vi "SP Sort Limit Points by Frequency.vi"(4 "Points":T1[](array[typedef])) -> (1 "Sorted Points":T1[](array[typedef]))   [LabVIEW 2011]
uses:
  TypeDefs/SP Limit Point.ctl
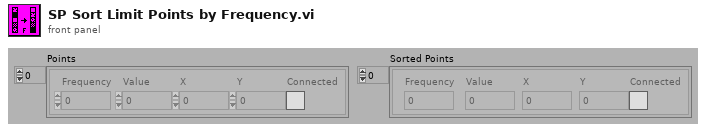
[diagram p1: front panel]
types:
  T1 = typedef "SP Limit Point.ctl" = cluster{"Frequency":dbl, "Value":dbl, "X":dbl, "Y":dbl, "Connected":bool}
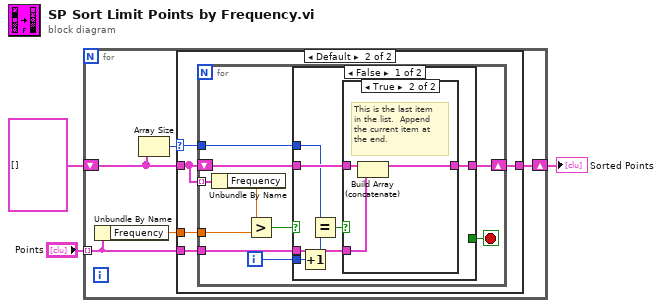
[diagram p0: block diagram]
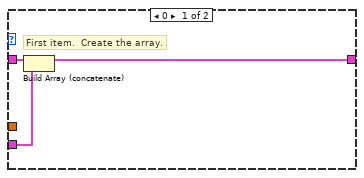
[diagram p2: hidden frame]
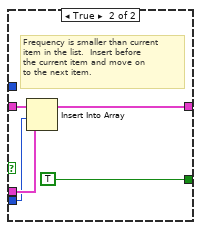
[diagram p4: hidden frame]
diagram:
  n1 = for {
    tunnel: "Points" -> [w6] mode=indexing
    shift-right: [w7] -> w2
    shift-left: T1[] [] ("Points") -> [w8]
    n2 = Unbundle By Name(w6) -> ("Frequency"=w5:dbl)
    n3 = Array Size(array=w8) -> (size(s)=w4:i32)
    n4 = case shown="Default" w4 {
      selector: w4 -> [_ w12]
      tunnel: w5 -> [_ w16]
      tunnel: w6 -> [w10 w15]
      tunnel: [w9 w14] -> w7
      tunnel: w8 -> [w11 w13]
      frame 0 {
        # "First item.  Create the array."
        n5 = Build Array (concatenate)(w11, w10) -> (w9:T1[])
      }
      frame Default {
        n6 = for {
          tunnel: w13 -> [w26] mode=indexing
          tunnel: w16 -> [w17]
          tunnel: w15 -> [w24]
          shift-right: [w22] -> w14
          shift-left: w13 -> [w23]
          tunnel: w12 -> [w19]
          i -> [w21]
          stop <- w20 stop-if-true
          n7 = Unbundle By Name(w26) -> ("Frequency"=w18:dbl)
          n8 = Greater?(x=w18, y=w17) -> (0:w25:bool)
          n9 = case shown="False" w25 {
            tunnel: [w28 w42] -> w22
            tunnel: [_ TRUE] -> w20
            tunnel: w24 -> [w30 w39]
            tunnel: w23 -> [w29 w40]
            tunnel: w21 -> [w32 w38]
            tunnel: w19 -> [w27 _]
            frame False {
              n10 = Increment(x=w32) -> (x+1=w33:i32)
              n11 = Equal?(x=w27, y=w33) -> (x = y?=w31:bool)
              n12 = case shown="True" w31 {
                tunnel: w29 -> [w34 w37]
                tunnel: w30 -> [_ w36]
                tunnel: [w34 w35] -> w28
                frame False {
                }
                frame True {
                  # "This is the last item\nin the list.  Append\nthe current item at \nthe end."
                  n13 = Build Array (concatenate)(w37, w36) -> (w35:T1[])
                }
              }
            }
            frame True {
              # "Frequency is smaller than current\nitem in the list.  Insert before\nthe current item and move on\nto the next item."
              n14 = Insert Into Array(array=w40, index=w38, new element=w39) -> (w42:T1[])
            }
          }
        }
      }
    }
  }
  "Sorted Points" <- w2
